vi "Team Selection UI.vi"(7 "Dev Team":refnum<class "Team.lvclass">) -> (1 "Cancelled":bool, 3 "Team":refnum<class "Team.lvclass">)   [LabVIEW 2020, in "SB App.lvlib" / "SB App.lvclass"]
uses:
  SB App.lvclass
  SquareBattle/Team/Team.lvclass
panel:
  out "Available Teams":refnum<class "Team.lvclass">[](array[class])
  in  "Cancel Button":bool
  in  "OK Button":bool
  in  "Selected Team":i32(listbox)
  # "Select Team to add to game:"
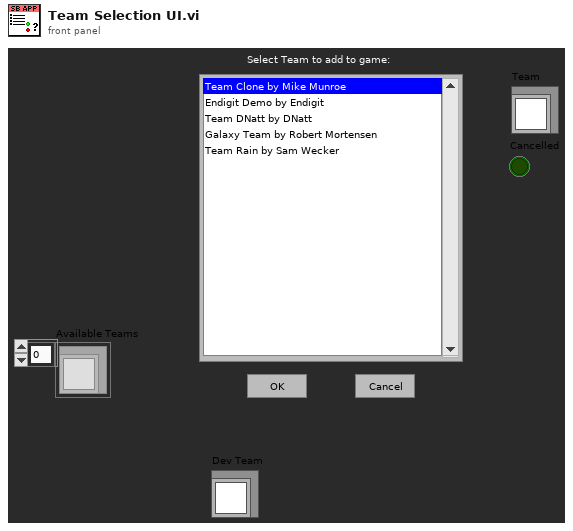
[diagram p1: front panel]
types:
  T1 = enum32{"Invalid", "Standard", "Closed", "Hidden", "Minimized", "Maximized"}
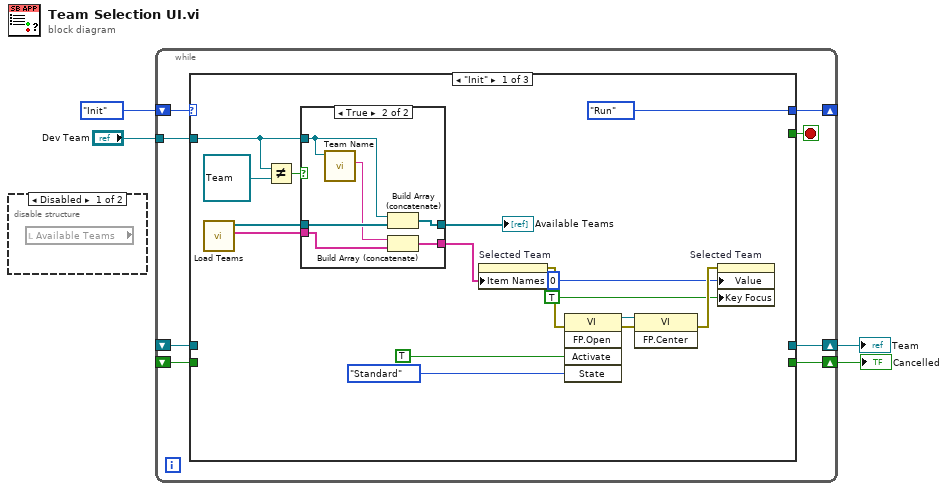
[diagram p0: block diagram]
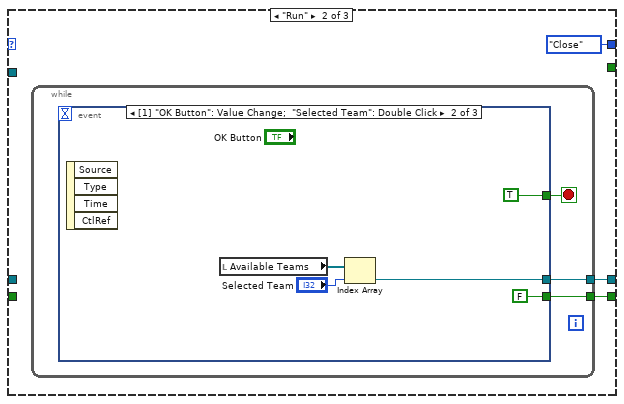
[diagram p4: hidden frame]
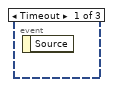
[diagram p5: hidden frame]
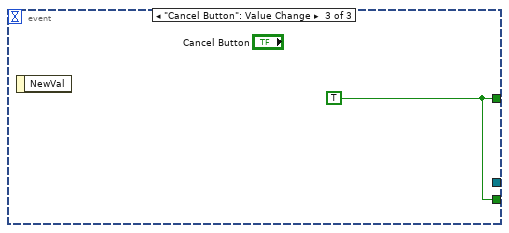
[diagram p6: hidden frame]
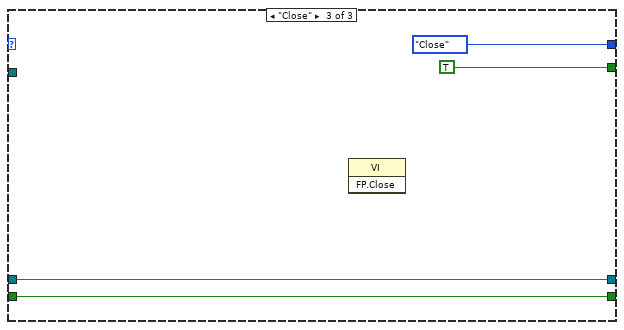
[diagram p7: hidden frame]
diagram:
  n1 = disable-structure shown="Disabled" {
    frame Disabled {
      n2 = local read "Available Teams"() -> ()  [unwired: 1 out]
    }
    frame Enabled {
    }
  }
  n3 = while {
    shift-right: [w11] -> _
    shift-left: enum16{"Init", "Run", "Close"}."Init" ("Basic UI State") -> [w12]
    shift-right: [w9] -> w3
    shift-left: _ -> [w8]
    shift-right: [w7] -> w2
    shift-left: _ -> [w6]
    tunnel: "Dev Team" -> [w5]
    stop <- w10 stop-if-true
    n4 = case shown="\"Init\"" w12 {
      tunnel: [enum16{"Init", "Run", "Close"}."Run" ("Basic UI State") enum16{"Init", "Run", "Close"}."Close" ("Basic UI State") enum16{"Init", "Run", "Close"}."Close" ("Basic UI State")] -> w11
      tunnel: [_ _ TRUE] -> w10
      tunnel: [_ w38 w50] -> w9
      tunnel: w8 -> [_ _ w50]
      tunnel: [_ w37 w49] -> w7
      tunnel: w6 -> [_ _ w49]
      tunnel: w5 -> [w16 _ _]
      frame "Init" {
        n5 = call "Load Teams.vi"() -> ("Names"=w15:string[], "Available Teams"=w18:refnum<class "Team.lvclass">[])  [unwired: 10 in]
        n6 = Not Equal?(x=w16, y=refnum<class "Team.lvclass"> refnum) -> (x != y?=w17:bool)
        n7 = case shown="True" w17 {
          tunnel: w18 -> [w30 w35]
          tunnel: w16 -> [_ w34]
          tunnel: w15 -> [w29 w36]
          tunnel: [w30 w32] -> w14
          tunnel: [w29 w31] -> w13
          frame False {
          }
          frame True {
            n8 = call-dynamic "Team Name.vi"("Team in"=w34) -> ("Team Name"=w33:string)  [unwired: 10 in]
            n9 = Build Array (concatenate)(w34, w35) -> (w32:refnum<class "Team.lvclass">[])
            n10 = Build Array (concatenate)(w33, w36) -> (w31:string[])
          }
        }
        "Available Teams" <- w14
        n11 = property on="Selected Team" class="LstBox (strict)"("Item Names"=w13) -> (error out=w23:errorcluster)  [unwired: 2 in, 1 out]
        n12 = invoke class="VI" method="FP.Open"(error in=w23, "Activate"=TRUE ("Activate?"), "State"=T1."Standard") -> (reference out=w24:refnum<vi>, error out=w22:errorcluster)  [unwired: 2 in, 3 out]
        n13 = invoke class="VI" method="FP.Center"(reference=w24, error in=w22) -> (error out=w28:errorcluster)  [unwired: 1 in, 2 out]
        n14 = property on="Selected Team" class="LstBox (strict)"(error in=w28, "Value"=0 ("Team"), "Key Focus"=TRUE) -> ()  [unwired: 1 in, 2 out]
      }
      frame "Run" {
        n15 = while {
          tunnel: [w42] -> w38
          tunnel: [w40] -> w37
          stop <- w41 stop-if-true
          n16 = event shown="[1] \"OK Button\": Value Change;  \"Selected Team\": Double Click" {
            selector: _ -> [_ _ _]
            dyn-events: _ -> [_ _ _]
            timeout: _ -> [_ _ _]
            tunnel: [_ w45 _] -> w42
            tunnel: [_ TRUE w48] -> w41
            tunnel: [_ FALSE w48] -> w40
            event Timeout {
              n17 = event-data() -> ()  [unwired: 1 in, 1 out]
            }
            event "OK Button": Value Change; "Selected Team": Double Click {
              n18 = event-data() -> ()  [unwired: 1 in, 4 out]
              n19 = local read "Available Teams"() -> (w47:refnum<class "Team.lvclass">[])
              n20 = Index Array(array=w47, index="Selected Team") -> (element=w45:refnum<class "Team.lvclass">)
            }
            event "Cancel Button": Value Change {
              w48 = TRUE
              n21 = event-data() -> ()  [unwired: 1 in, 1 out]
            }
          }
        }
      }
      frame "Close" {
        n22 = invoke class="VI" method="FP.Close"() -> ()  [unwired: 3 in, 3 out]
      }
    }
  }
  "Team" <- w3
  "Cancelled" <- w2
